vi "Quick Usb Set Timeout.vi"(8 "error in (no error)":errorcluster, 10 "timeOut":u32, 11 "hDevice":u32) -> (0 "error out":errorcluster, 2 "function return":i32, 3 "hDevice out":u32)   [LabVIEW 2011, in "QuickUSB.lvlib"]
doc: "QUSBLIB QRETURN QuickUsbSetTimeout(\n QHANDLE hDevice,\n QULONG timeOut\n);"
uses:
  QuickUSB.lvlib
  QuickUSB.dll
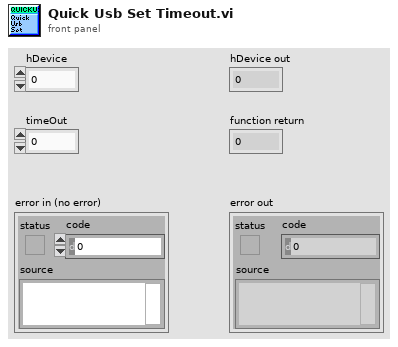
[diagram p1: front panel]
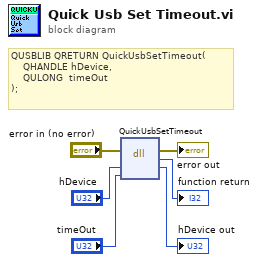
[diagram p0: block diagram]
diagram:
  # "QUSBLIB QRETURN QuickUsbSetTimeout(\n    QHANDLE hDevice,\n    QULONG  timeOut\n);"
  n1 = dll-call lib="C:/QuickUSB/QuickUSB.*" fn="QuickUsbSetTimeout"(error in="error in (no error)", "hDevice"="hDevice", "timeOut"="timeOut") -> (error out=→"error out":errorcluster, →"function return":i32, "hDevice"=→"hDevice out":u32)  [unwired: 3 in, 1 out]
